vi "Write configuration.vi"(8 "error in":errorcluster, 10 "configuration in":refnum<class "NISE_CEF_serializable configuration.lvclass">, 11 "Scan Engine editor node in":refnum<class "Scan Engine editor node.lvclass">) -> (0 "error out":errorcluster, 3 "Scan Engine editor node out":refnum<class "Scan Engine editor node.lvclass">)   [LabVIEW 2013, in "Scan Engine editor node.lvclass"]
uses:
  Scan Engine editor node.lvclass
  <vilib>/NI/Configuration Framework/serializable configuration/NISE_CEF_serializable configuration.lvclass
  <vilib>/NI/TBM Modules/variable/module/configuration/Scan Engine configuration.lvclass
  Scan Engine editor node.lvclass/Scan Engine editor node.ctl
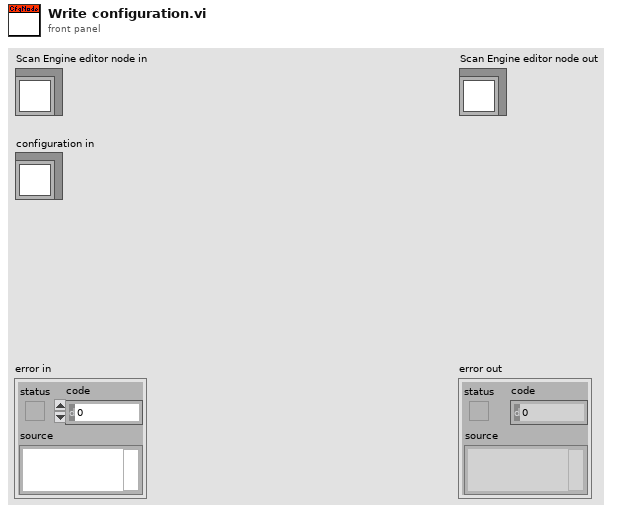
[diagram p1: front panel]
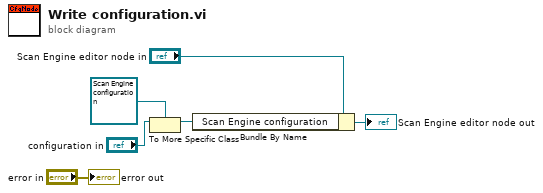
[diagram p0: block diagram]
diagram:
  n1 = To More Specific Class(target class=refnum<class "Scan Engine configuration.lvclass"> refnum ("Scan Engine configuration"), reference="configuration in") -> (specific class reference=w4:refnum<class "Scan Engine configuration.lvclass">)  [unwired: 1 in, 1 out]
  n2 = Bundle By Name(cluster="Scan Engine editor node in", "Scan Engine configuration"=w4) -> (→"Scan Engine editor node out":refnum<class "Scan Engine editor node.lvclass">)
  "error out" <- "error in"
